vi "Locate Spark with Optimizer.vi"(0 "Channel Data":dbl[][](array[numeric]), 1 "Search Channel":i32, 2 "Sampling Rate":i32=500000, 5 "Min Spark Duration (s)":dbl=0.01, 7 "Wavefront Window Duration (s)":dbl=0.0006, 9 "RF Hammer Duration (s)":dbl=0.0002, 11 "error in (no error)":errorcluster, 13 "Sensor Configuration":i32[](array[numeric])) -> (4 "Coordinates (s)":cluster{sgl, sgl, sgl}, 6 "Normalized Diameter":dbl, 8 "Normalized Length":dbl, 10 "Chi^2":dbl, 15 "error out":errorcluster)   [LabVIEW 2012]
uses:
  <vilib>/gmath/NumericalOptimization/cno_bounds.ctl
  <vilib>/gmath/NI_Gmath.lvlib
panel:
  out "Search Channel Signal":dbl[](graph)
  out "coordinates":cluster{dbl, dbl, dbl}
  out "Wavefront Times":dbl[](array[numeric])
  out "coordinates_prime":T1
  # "x"
  # "y"
  # "z"
  # "Upstream"
  # "0 Degrees"
  # "90 Degrees"
  # "180 Degrees"
  # "270 Degrees"
  # "Downstream"
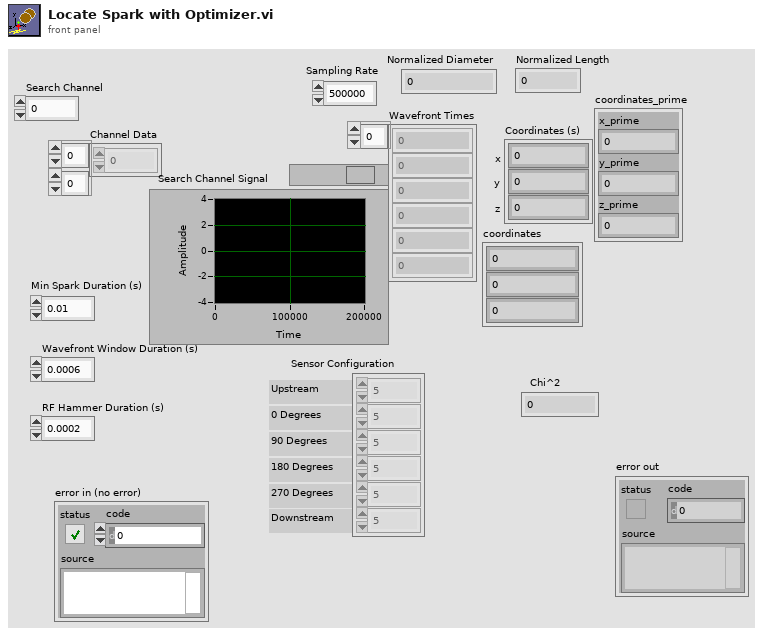
[diagram p1: front panel]
types:
  T1 = cluster{"x_prime":dbl, "y_prime":dbl, "z_prime":dbl}
  T2 = typedef "NI_Gmath.lvlib/cno_bounds.ctl" = cluster{"X minimum":dbl[], "X maximum":dbl[], "inequality constraint minimum":dbl[], "inequality constraint maximum":dbl[]}
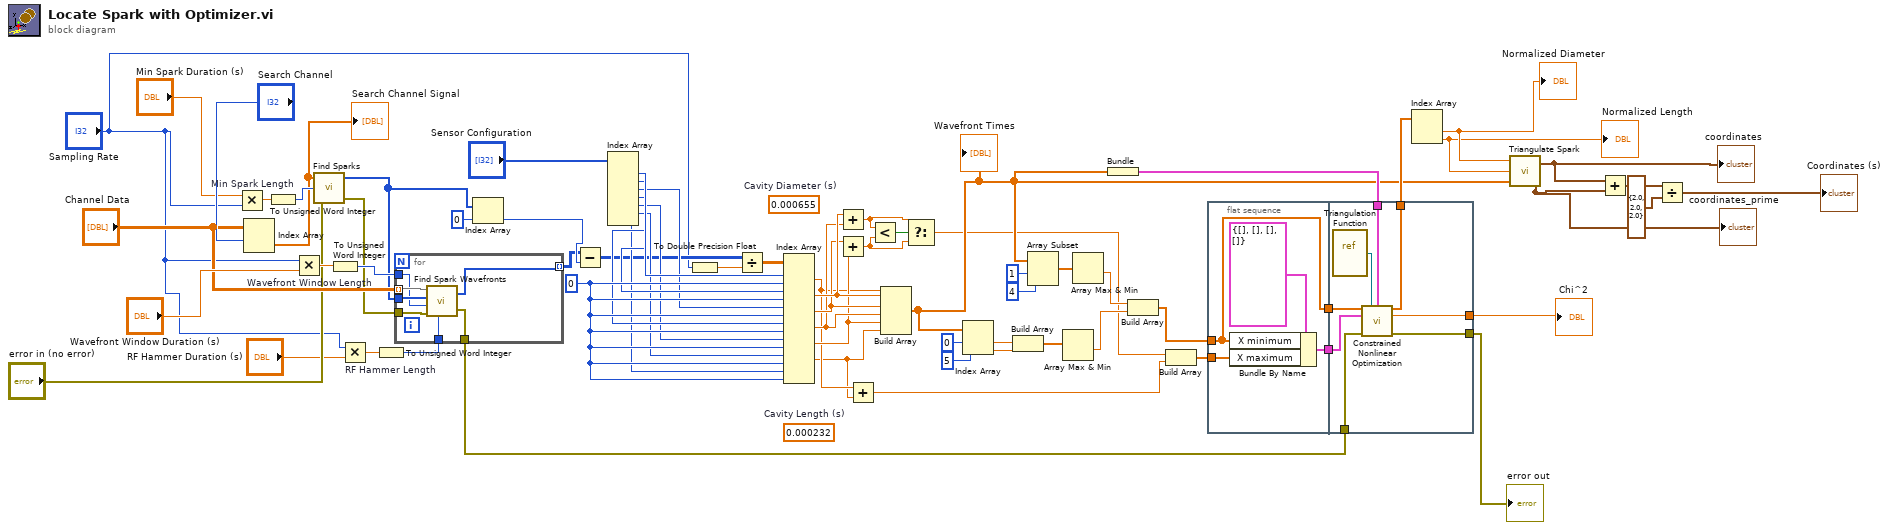
[diagram p0: block diagram]
diagram:
  (unwired) 0.000655  # Cavity Diameter (s)
  (unwired) 0.000232  # Cavity Length (s)
  w62 = 0 ("disabled index (col)")
  n1 = Multiply "Min Spark Length"(x="Min Spark Duration (s)", y="Sampling Rate") -> (x*y=w67:dbl)
  n2 = Index Array(array="Channel Data", index (row)="Search Channel") -> (element=w1:dbl[])  [unwired: 1 in]
  "Search Channel Signal" <- w1
  n3 = To Unsigned Word Integer(number=w67) -> (unsigned 16bit integer=w39:u16)
  n4 = Multiply "Wavefront Window Length"(x="Sampling Rate", y="Wavefront Window Duration (s)") -> (x*y=w65:dbl)
  n5 = call <userlib>:"Find Sparks.vi"("error in (no error)"="error in (no error)", "Min Spark Length"=w39, "Waveform"=w1) -> ("error out"=w37:errorcluster, "Spark Indicies"=w38:i32[])  [unwired: 1 in]
  n6 = To Unsigned Word Integer(number=w65) -> (unsigned 16bit integer=w64:u16)
  n7 = Multiply "RF Hammer Length"(x="Sampling Rate", y="RF Hammer Duration (s)") -> (x*y=w32:dbl)
  n8 = To Unsigned Word Integer(number=w32) -> (unsigned 16bit integer=w31:u16)
  n9 = for {
    tunnel: w38 -> [w76]
    tunnel: w64 -> [w74]
    tunnel: [w71] -> w49 mode=indexing
    tunnel: "Channel Data" -> [w75] mode=indexing
    tunnel: w37 -> [w73]
    tunnel: [w72] -> w36
    tunnel: w31 -> [w70]
    n10 = call <userlib>:"Find Spark Wavefronts.vi"("RF Hammer Length"=w70, "error in (no error)"=w73, "Window Length"=w74, "Spark Indicies"=w76, "Waveform"=w75) -> ("error out"=w72:errorcluster, "Wavefront Indicies"=w71:i32[])  [unwired: 1 in]
  }
  n11 = Index Array(array=w38, index=0) -> (element=w53:i32)
  n12 = Subtract(x=w49, y=w53) -> (x-y=w52:i32[][])
  n13 = Index Array(array="Sensor Configuration") -> (element #1=w61:i32, element #2=w60:i32, element #3=w59:i32, element #4=w58:i32, element #5=w57:i32, element #6=w56:i32, element #7=w55:i32)  [unwired: 7 in]
  n14 = To Double Precision Float(number="Sampling Rate") -> (double precision float=w51:dbl)
  n15 = Divide(x=w52, y=w51) -> (x/y=w50:dbl[][])
  n16 = Index Array(array=w50, index (row) #1=w61, index (col) #1=w62, index (row) #2=w60, index (col) #2=w62, index (row) #3=w59, index (col) #3=w62, index (row) #4=w58, index (col) #4=w62, index (row) #5=w57, index (col) #5=w62, index (row) #6=w56, index (col) #6=w62, index (row) #7=w55, index (col) #7=w62) -> (element #1=w9:dbl, element #2=w18:dbl, element #3=w17:dbl, element #4=w16:dbl, element #5=w15:dbl, element #6=w8:dbl)  [unwired: 1 out]
  n17 = Add(x=w18, y=w16) -> (x+y=w47:dbl)
  n18 = Add(x=w17, y=w15) -> (x+y=w46:dbl)
  n19 = Add(x=w9, y=w8) -> (x+y=w7:dbl)
  n20 = Less?(x=w47, y=w46) -> (x < y?=w48:bool)
  n21 = Build Array(w9, w18, w17, w16, w15, w8) -> (w12:dbl[])
  "Wavefront Times" <- w12
  n22 = Select(t=w47, s=w48, f=w46) -> (s? t:f=w10:dbl)
  n23 = Index Array(array=w12, index #1=0 ("index"), index #2=5 ("index")) -> (element #1=w25:dbl, element #2=w24:dbl)
  n24 = Build Array(w25, w24) -> (w22:dbl[])
  n25 = Array Subset(array=w12, index=1, length=4) -> (w23:dbl[])
  n26 = Array Max & Min(array=w22) -> (min value=w20:dbl)  [unwired: 3 out]
  n27 = Array Max & Min(array=w23) -> (min value=w21:dbl)  [unwired: 3 out]
  n28 = Bundle(w12) -> (w43:cluster{dbl[]})  [unwired: 1 in]
  n29 = Build Array(w21, w20) -> (w19:dbl[])
  n30 = Build Array(w10, w7) -> (w44:dbl[])
  n31 = flat-sequence {
    tunnel: w44 -> [w78]
    tunnel: [w79] -> w45
    tunnel: w19 -> [w77]
    tunnel: [w77] -> w11
    tunnel: w45 -> [w87]
    tunnel: w43 -> [w86]
    tunnel: [w85] -> w42
    tunnel: [w84] -> w40
    tunnel: w36 -> [w83]
    tunnel: [w82] -> w35
    tunnel: w11 -> [w81]
    frame #0 {
      n32 = Bundle By Name(cluster=T2 {"X minimum"=[], "X maximum"=[], "inequality constraint minimum"=[], "inequality constraint maximum"=[]} ("bounds"), "X minimum"=w77, "X maximum"=w78) -> (w79:T2)
    }
    frame #1 {
      n33 = vi-ref <userlib>:"Triangulation Function.vi"() -> (w88:refnum<vi>)
      n34 = call <vilib>:"Constrained Nonlinear Optimization.vi"("start"=w81, "objective and constraint function"=w88, "function data"=w86, "bounds"=w87, "error in (no error)"=w83) -> ("minimum"=w85:dbl[], "f(minimum)"=w84:dbl, "error out"=w82:errorcluster)  [unwired: 6 in, 2 out]
    }
  }
  n35 = Index Array(array=w42) -> (element #1=w14:dbl, element #2=w13:dbl)  [unwired: 2 in]
  "Normalized Diameter" <- w14
  "Normalized Length" <- w13
  n36 = call <userlib>:"Triangulate Spark.vi"("timings"=w12, "cavity length (s)"=w13, "cavity diameter (s)"=w14) -> ("coordinates_prime"=w5:T1, "coordinates"=w3:cluster{"x":dbl, "y":dbl, "z":dbl})  [unwired: 1 in]
  "coordinates_prime" <- w5
  "coordinates" <- w3
  n37 = Add(x=w3, y=w5) -> (x+y=w6:cluster{dbl, dbl, dbl})
  n38 = Divide(x=w6, y=cluster{dbl, dbl, dbl} {2.0, 2.0, 2.0}) -> (x/y=→"Coordinates (s)":cluster{dbl, dbl, dbl})
  "Chi^2" <- w40
  "error out" <- w35
